vi "禹山溶解氧_获取温度和测量值.vi"(5 "大气压补偿":dbl=1.0, 7 "盐度补偿":dbl, 8 "error in (no error)":errorcluster caption="错误输入（无错误）", 11 "MB_Serial session in":refnum<class "MB_Master_Serial.lvclass">) -> (0 "error out":errorcluster caption="错误输出", 2 "输出值":cluster{"温度测量值":sgl, "DO%":sgl, "DOmg/L":sgl}, 3 "MB_Serial session out":refnum<class "MB_Master_Serial.lvclass">)   [LabVIEW 2016, in "斯坦道多参数.lvlib"]
uses:
  <vilib>/Plasmionique/MB Master/MB_Master_Serial/MB_Master_Serial.lvclass
  C:/Program Files (x86)/National Instruments/LabVIEW 2016/vi.lib/Plasmionique/MB Master/MB_Master/MB_Master.lvclass
  <vilib>/Plasmionique/MB Master/MB Master.lvlib
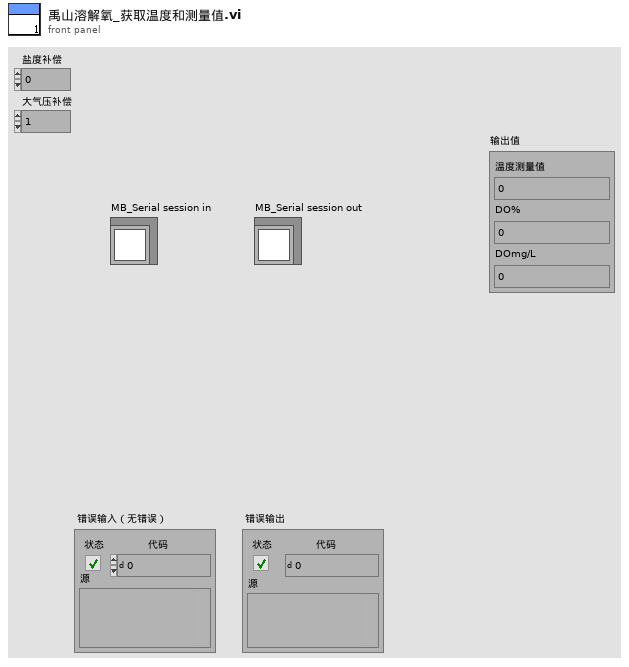
[diagram p1: front panel]
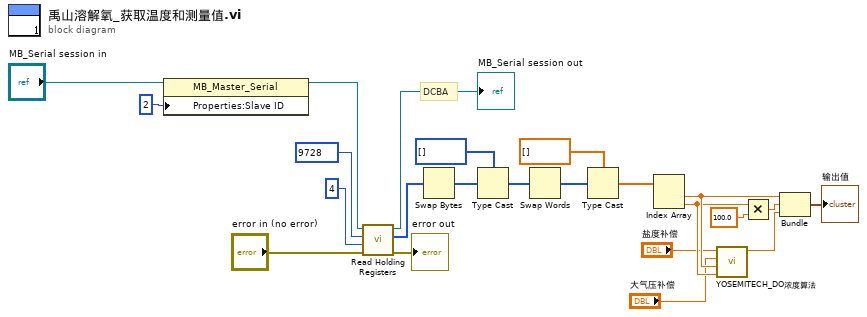
[diagram p0: block diagram]
diagram:
  # "DCBA"
  n1 = property class="MB_Master_Serial"(reference="MB_Serial session in", "Properties:Slave ID"=u16 2 ("y")) -> (reference out=w14:refnum<class "MB_Master_Serial.lvclass">)  [unwired: 1 in, 1 out]
  n2 = call <vilib>:"Read Holding Registers.vi"("error in (no error)"="error in (no error)", "quantity"=u16 4, "starting address"=u16 9728, "MB session in"=w14) -> ("error out"=→"error out":errorcluster, "Registers"=w9:u16[], "MB session out"=→"MB_Serial session out":refnum<class "MB_Master_Serial.lvclass">)  [unwired: 5 in]
  n3 = Swap Bytes(anything=w9) -> (byte swapped=w8:u16[])
  n4 = Type Cast(type=u32[] [] ("数组 2"), x=w8) -> (*(type *) &x=w18:u32[])
  n5 = Swap Words(1:w18) -> (0:w20:u32[])
  n6 = Type Cast(type=sgl[] [] ("数组 2"), x=w20) -> (*(type *) &x=w16:sgl[])
  n7 = Index Array(array=w16) -> (element #1=w7:sgl, element #2=w6:sgl)  [unwired: 2 in]
  n8 = call "YOSEMITECH_DO浓度算法.vi"("溶解氧饱和度值"=w6, "水温"=w7, "大气压补偿"="大气压补偿", "盐度补偿"="盐度补偿") -> ("DataDo_mgL"=w5:dbl)  [unwired: 7 in]
  n9 = Multiply(x=w6, y=sgl 100.0) -> (x*y=w2:sgl)
  n10 = Bundle("数值"=w7, w2, "DataDo_mgL"=w5) -> (→"输出值":cluster{"数值":sgl, sgl, "DataDo_mgL":dbl})  [unwired: 1 in]
